vi "Send Status.vi"(8 "error in (no error)":errorcluster, 9 "Name":string, 10 "Status":string, 11 "UI Main in":refnum<class "UI Main.lvclass">) -> (0 "error out":errorcluster, 3 "UI Main out":refnum<class "UI Main.lvclass">)   [LabVIEW 2021, in "UI Main.lvlib" / "UI Main.lvclass"]
uses:
  UI Main.lvclass
  UI Main.lvclass/UI Main.ctl
  UI Status/UI Status Messages/Update Status Msg/Update Status Msg.lvclass/Update Status Msg.ctl
  <vilib>/ActorFramework/Message Enqueuer/Message Enqueuer.lvclass/Message Enqueuer.ctl
  <vilib>/ActorFramework/Message Enqueuer/Enqueue.vi
  UI Status/UI Status Messages/Update Status Msg/Update Status Msg.lvclass
  C:/Program Files (x86)/National Instruments/LabVIEW 2021/vi.lib/ActorFramework/Message/Message.lvclass
  <vilib>/ActorFramework/Message Priority Queue/Priority Enqueue.vi
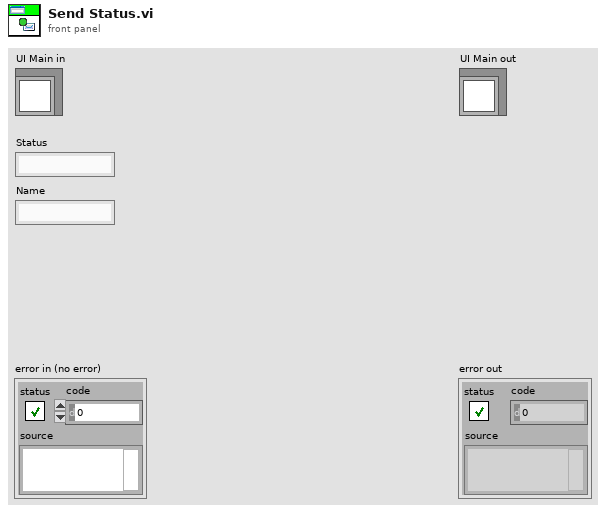
[diagram p1: front panel]
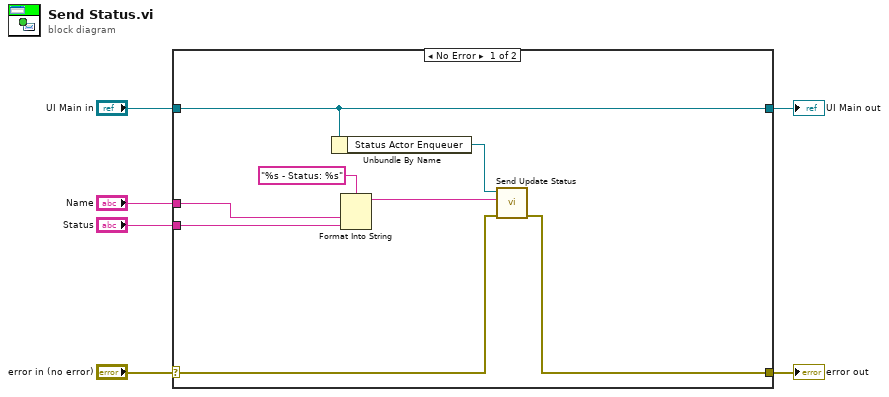
[diagram p0: block diagram]
diagram:
  n1 = case shown="No Error" "error in (no error)" {
    selector: "error in (no error)" -> [w8 w16]
    tunnel: [w7 w16] -> w5
    tunnel: [w14 w15] -> w3
    tunnel: "UI Main in" -> [w14 w15]
    tunnel: "Status" -> [w10 _]
    tunnel: "Name" -> [w11 _]
    frame No Error {
      n2 = Unbundle By Name(w14) -> ("Status Actor Enqueuer"=w13:refnum<class "Message Enqueuer.lvclass">)
      n3 = Format Into String(format string="%s - Status: %s", w11, w10) -> (resulting string=w9:string)  [unwired: 2 in, 1 out]
      n4 = call "Send Update Status.vi"("error in (no error)"=w8, "Status"=w9, "Message Enqueuer"=w13) -> ("error out"=w7:errorcluster)  [unwired: 7 in, 1 out]
    }
    frame Error {
    }
  }
  "error out" <- w5
  "UI Main out" <- w3
